vi "PlotMieCurve.vi"(3 "refractive index, imaginary":sgl=0.1 step=0.01 format="%.3f", 4 "refractive index, real":sgl=1.3 step=0.01 format="%.3f", 5 "Use Extinction Factor":bool, 6 "Extinction ExtinctionUncertainity Size parameter and Number ofS sizes":T1={"Extinction"=[], "Extinction Uncertainty"=[], "Size parameters"=[], "Number ofSizes"=0.0, "GeometricCrossSection"=[], "Wave Length"=0.0, "SMPS Sizes"=[], "Concentration"=[], "Double Charge Correction"=FALSE, "Extincation Factor"=1.0, "Diameter Factor"=1.0, "Diameter Offset"=0.0, "Extinction Factor Flag"=FALSE, "Diameter Factor Flag"=FALSE, "Diameter Offset Flag"=FALSE, "Sizes"=[], "ExtinctionOrAbsorptionOrScattering"=0} {"ExtinctionOrAbsorptionOrScattering" scale=0.0..2.0}) -> (0 "Mie Results In Size Parameters":sgl[](array[numeric]), 1 "Size parameters":dbl[](array[numeric]), 2 "Extinction Crosssections":dbl[](array[numeric]))   [LabVIEW 2011]
uses:
  BaesDataTypeDefinition.ctl
  <vilib>/imath/engines/lvmath2/RunTimeEngine/ErrorHandling/NIMS_Finalize Error.vi
  <vilib>/imath/engines/lvmath2/RunTimeEngine/Managers/WorkSpace/UID Generator.vi
  <vilib>/imath/engines/lvmath2/RunTimeEngine/Managers/SymbolTable/Clear UID.vi
  <vilib>/imath/engines/lvmath2/RunTimeEngine/NodeEndStatement/NIMS_NodeEndStatement_Output.vi
  <instcachedir>/0/NIMS_NodeEndStatement_Output_53EC0D466D134D7ABD903AC30B43404B.lvgen/NIMS_NodeEndStatement_Output_53EC0D466D134D7ABD903AC30B43404B_005.vi
  <vilib>/imath/engines/lvmath2/RunTimeEngine/RunTimeType/NIMS_RunTimeType_From StrictType (excl LVString).vi
  <instcachedir>/0/NIMS_RunTimeType_From StrictType (excl LVString)_46AE8B54A11948F0BCCEB8091EE7AA4C.lvgen/NIMS_RunTimeType_From StrictType (excl LVString)_46AE8B54A11948F0BCCEB8091EE7AA4C_000.vi
  <vilib>/imath/engines/lvmath2/RunTimeEngine/LocalVariableDefStatement/MC_LocalVariableDefStatement_Display.vi
  <vilib>/imath/engines/lvmath2/RunTimeEngine/BuiltInFunctions/max/1 input/NIMS_max(RV).vi
  <instcachedir>/0/NIMS_max(RV)_237633DB1D604D5BA7001287DF3C7957.lvgen/NIMS_max(RV)_237633DB1D604D5BA7001287DF3C7957_000.vi
  <vilib>/imath/engines/lvmath2/RunTimeEngine/BuiltInFunctions/min/1 input/NIMS_min(RV).vi
  <instcachedir>/0/NIMS_min(RV)_EE2DD3E2888846108C5160A664B67832.lvgen/NIMS_min(RV)_EE2DD3E2888846108C5160A664B67832_000.vi
  <vilib>/imath/engines/lvmath2/RunTimeEngine/RangeToken/NIMS_Range.vi
  <instcachedir>/0/NIMS_Range_0B7635FB69F84E19AA68E7FF959DF37C.lvgen/NIMS_Range_0B7635FB69F84E19AA68E7FF959DF37C_001.vi
  <vilib>/imathl/engines/lvmath/Functions/Error Handling/Create Error.vi
  mie2.dll
  <vilib>/imath/engines/lvmath2/RunTimeEngine/Managers/SymbolTable/NIMS_WorkSpace.lvlib
panel:
  out "Numeric":i32
  out "totalscatter 3":sgl=3.7788873
  out "backscatter 3":sgl=8.098428
  out "<cos(theta)> 4":sgl=0.19839454
  out "extinction 3":sgl=1.6240653
  out "NewGeometricCrossSection":dbl[](array[numeric])
  in  "angles (will compute\n2*angles-1 points from\n0...180 degrees)":u32=2
  out "totalscatter 2":sgl=3.7788873
  out "backscatter 2":sgl=8.098428
  out "<cos(theta)> 3":sgl=0.19839454
  out "extinction 2":sgl=1.6240653
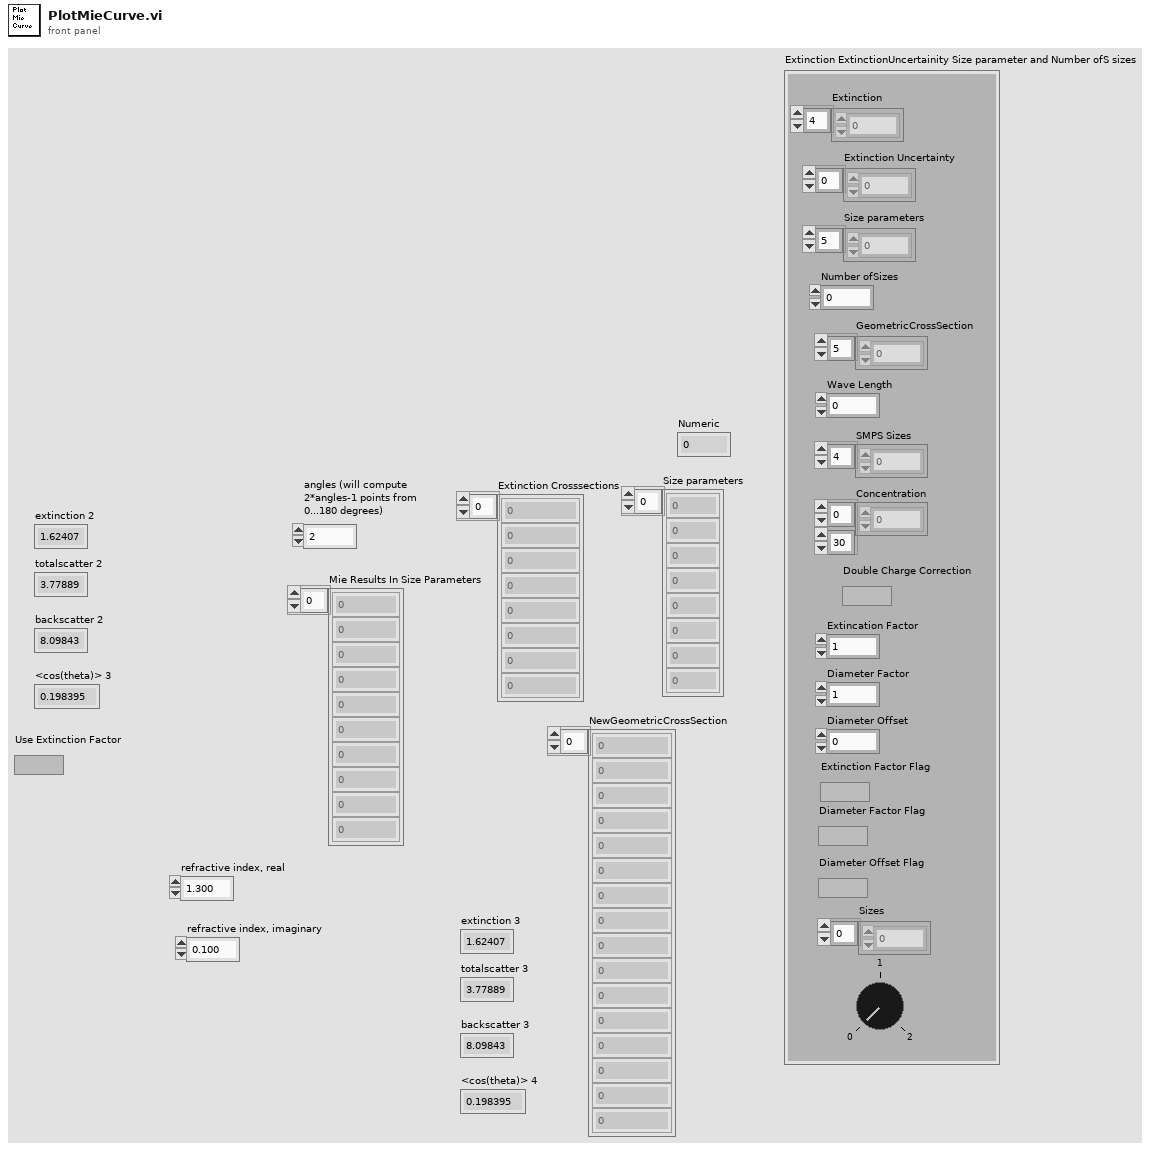
[diagram p1: front panel]
types:
  T1 = typedef "BaesDataTypeDefinition.ctl" = cluster{"Extinction":dbl[], "Extinction Uncertainty":dbl[], "Size parameters":dbl[], "Number ofSizes":dbl, "GeometricCrossSection":dbl[], "Wave Length":dbl, "SMPS Sizes":dbl[], "Concentration":dbl[][], "Double Charge Correction":bool, "Extincation Factor":dbl, "Diameter Factor":dbl, "Diameter Offset":dbl, "Extinction Factor Flag":bool, "Diameter Factor Flag":bool, "Diameter Offset Flag":bool, "Sizes":dbl[], "ExtinctionOrAbsorptionOrScattering":i8}
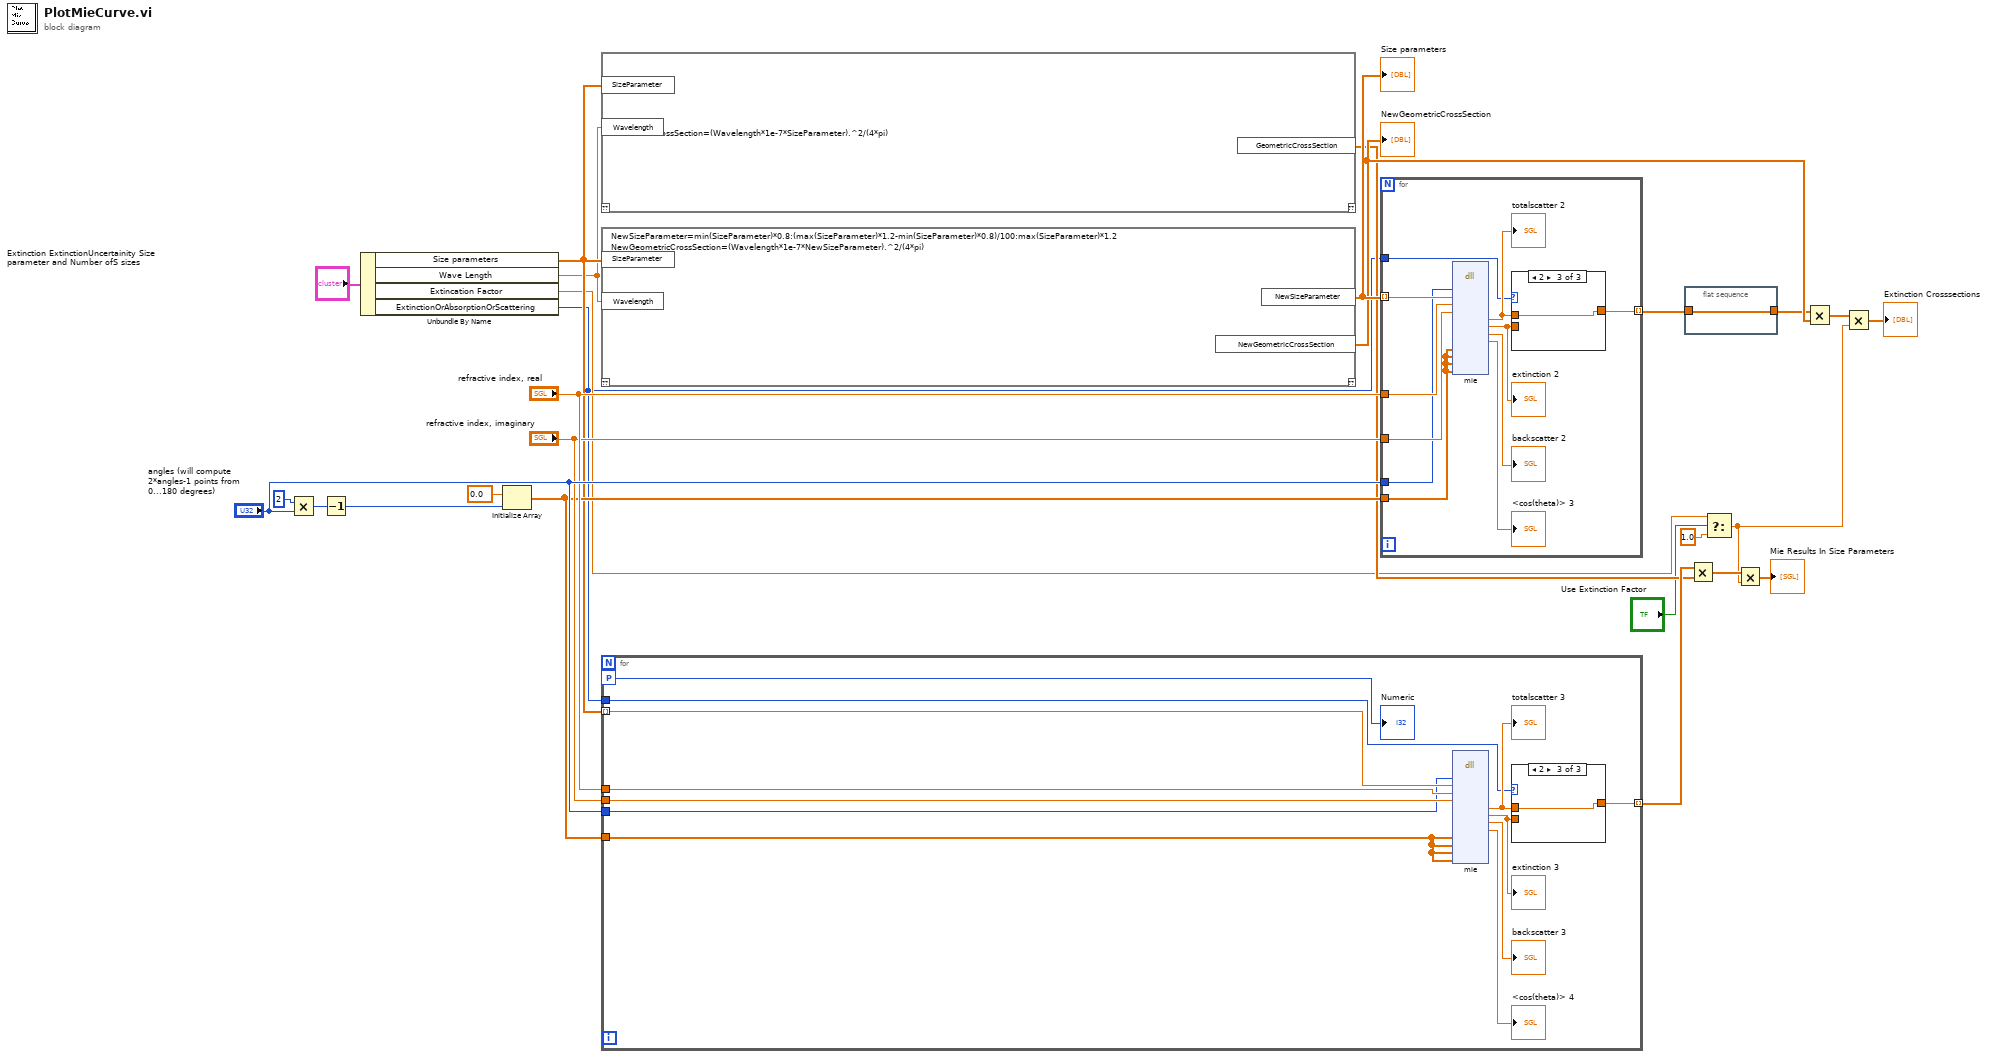
[diagram p0: block diagram]
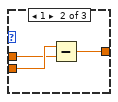
[diagram p3: hidden frame]
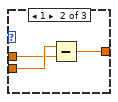
[diagram p5: hidden frame]
diagram:
  n1 = Multiply(x=u32 2, y="angles (will compute\n2*angles-1 points from\n0...180 degrees)") -> (x*y=w26:u32)
  n2 = Decrement(x=w26) -> (x-1=w22:u32)
  n3 = Unbundle By Name("Extinction ExtinctionUncertainity Size parameter and Number ofS sizes") -> ("Size parameters"=w12:dbl[], "Wave Length"=w11:dbl, "Extincation Factor"=w5:dbl, "ExtinctionOrAbsorptionOrScattering"=w1:i8)
  n4 = Initialize Array(sgl 0.0, w22) -> (w14:sgl[])
  n5 = mathscript code="GeometricCrossSection=(Wavelength*1e-7*SizeParameter).^2/(4*pi)"("SizeParameter"=w12, "Wavelength"=w11) -> ("GeometricCrossSection"=w10:dbl[])  [unwired: 1 in, 1 out]
  n6 = mathscript code="NewSizeParameter=min(SizeParameter)*0.8:(max(SizeParameter)*1.2-min(SizeParameter)*0.8)/100:max(SizeParameter)*1.2\nNewGeometricCrossSection=(Wavelength*1e-7*NewSizeParameter).^2/(4*pi)"("SizeParameter"=w12, "Wavelength"=w11) -> ("NewSizeParameter"=w21:dbl[], "NewGeometricCrossSection"=w20:dbl[])  [unwired: 1 in, 1 out]
  "Size parameters" <- w21
  "NewGeometricCrossSection" <- w20
  n7 = for {
    tunnel: w14 -> [w36]
    tunnel: [w29] -> w13 mode=indexing
    tunnel: "refractive index, real" -> [w35]
    tunnel: "refractive index, imaginary" -> [w34]
    tunnel: w12 -> [w33] mode=indexing
    tunnel: "angles (will compute\n2*angles-1 points from\n0...180 degrees)" -> [w32]
    workers-P: _ -> [w31]
    tunnel: w1 -> [w27]
    n8 = dll-call lib="Z:/Dropbox/Lior Segev/Lior Segev Projects/RI retrieval in Labview/NewCheckout/mie2.dll" fn="mie"("angles"=w32, "x"=w33, "r"=w35, "i"=w34, "spol_real"=w36, "spol_imaginary"=w36, "ppol_real"=w36, "ppol_imaginary"=w36) -> ("totalscatter"=w28:sgl, "extinction"=w30:sgl, "backscatter"=→"backscatter 3":sgl, "<cos(theta)>"=→"<cos(theta)> 4":sgl)  [unwired: 16 in, 2 out]
    "totalscatter 3" <- w28
    "extinction 3" <- w30
    n9 = case shown="2" w27 {
      tunnel: w30 -> [w39 w42 _]
      tunnel: [w39 w40 w43] -> w29
      tunnel: w28 -> [_ w41 w43]
      frame 0, Default {
      }
      frame 1 {
        n10 = Subtract(x=w42, y=w41) -> (x-y=w40:sgl)
      }
      frame 2 {
      }
    }
    "Numeric" <- w31
  }
  n11 = for {
    tunnel: w14 -> [w52]
    tunnel: [w46] -> w2 mode=indexing
    tunnel: "refractive index, real" -> [w51]
    tunnel: "refractive index, imaginary" -> [w50]
    tunnel: w21 -> [w49] mode=indexing
    tunnel: "angles (will compute\n2*angles-1 points from\n0...180 degrees)" -> [w48]
    tunnel: w1 -> [w44]
    n12 = dll-call lib="Z:/Dropbox/Lior Segev/Lior Segev Projects/RI retrieval in Labview/NewCheckout/mie2.dll" fn="mie"("angles"=w48, "x"=w49, "r"=w51, "i"=w50, "spol_real"=w52, "spol_imaginary"=w52, "ppol_real"=w52, "ppol_imaginary"=w52) -> ("totalscatter"=w45:sgl, "extinction"=w47:sgl, "backscatter"=→"backscatter 2":sgl, "<cos(theta)>"=→"<cos(theta)> 3":sgl)  [unwired: 16 in, 2 out]
    "totalscatter 2" <- w45
    "extinction 2" <- w47
    n13 = case shown="2" w44 {
      tunnel: w47 -> [w55 w58 _]
      tunnel: [w55 w56 w59] -> w46
      tunnel: w45 -> [_ w57 w59]
      frame 0, Default {
      }
      frame 1 {
        n14 = Subtract(x=w58, y=w57) -> (x-y=w56:sgl)
      }
      frame 2 {
      }
    }
  }
  n15 = flat-sequence {
    tunnel: [w60] -> w3
    tunnel: w2 -> [w60]
    frame #0 {
    }
  }
  n16 = Multiply(x=w13, y=w10) -> (x*y=w9:dbl[])
  n17 = Select(t=w5, s="Use Extinction Factor", f=1.0) -> (s? t:f=w4:dbl)
  n18 = Multiply(x=w9, y=w4) -> (x*y=→"Mie Results In Size Parameters":dbl[])
  n19 = Multiply(x=w3, y=w20) -> (x*y=w19:dbl[])
  n20 = Multiply(x=w19, y=w4) -> (x*y=→"Extinction Crosssections":dbl[])
